vi "Recieve Timer Tick.vi"(8 "error in (no error)":errorcluster, 10 "Time Stamp Control":timestamp, 11 "Measurement Timer in":refnum<class "Measurement Timer.lvclass">) -> (0 "error out":errorcluster, 3 "Measurement Timer out":refnum<class "Measurement Timer.lvclass">)   [LabVIEW 2015, in "Measurement Timer.lvclass"]
uses:
  Measurement Timer.lvclass
  Measurement Timer.lvclass/Measurement Timer.ctl
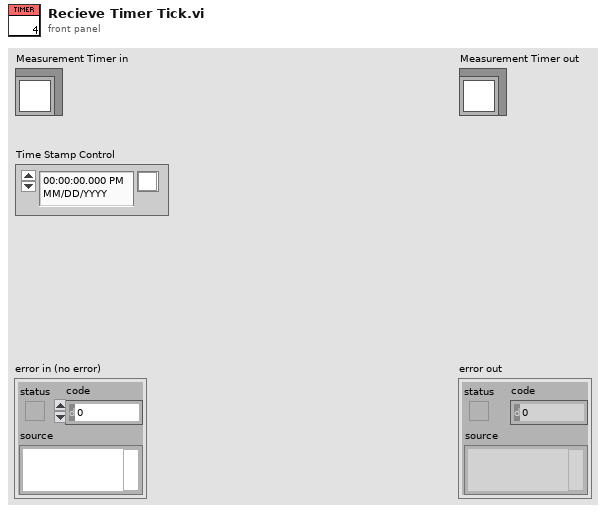
[diagram p1: front panel]
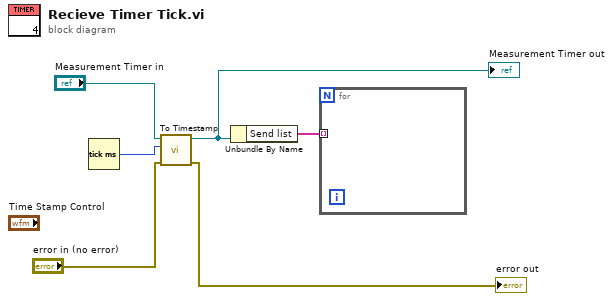
[diagram p0: block diagram]
diagram:
  n1 = Tick Count (ms)() -> (millisecond timer value=w5:u32)
  n2 = call-dynamic "To Timestamp.vi"("error in (no error)"="error in (no error)", "milliseconds timer value"=w5, "Measurement Timer in"="Measurement Timer in") -> ("error out"=→"error out":errorcluster, "Measurement Timer out"=w2:refnum<class "Measurement Timer.lvclass">)  [unwired: 6 in, 1 out]
  "Measurement Timer out" <- w2
  n3 = Unbundle By Name(w2) -> ("Send list"=w3:string[])
  n4 = for {
    tunnel: w3 -> [_] mode=indexing
  }
